vi "Read_BIn.vi"(0 "Refnum in":refnum<k21>, 5 "error in (no error)":errorcluster) -> (14 "Refnum out":refnum<k21>, 15 "Estados":bool[](array[boolean]), 19 "error out":errorcluster)   [LabVIEW 2013]
uses:
  <vilib>/DAQmx/read.llb/DAQmx Read (Digital U32 1Chan 1Samp).vi
  <vilib>/DAQmx/miscellaneous.llb/DAQmx Fill In Error Info.vi
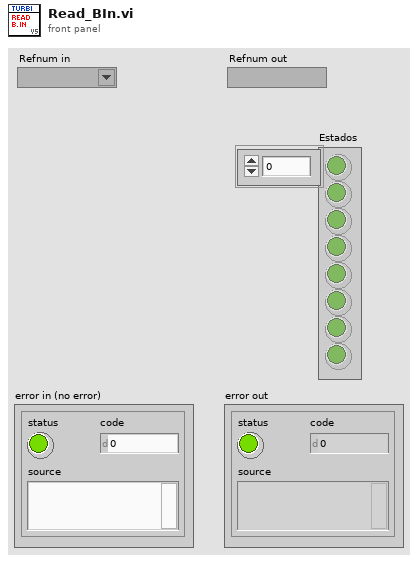
[diagram p1: front panel]
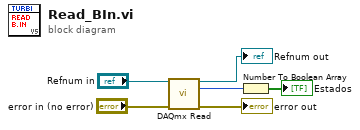
[diagram p0: block diagram]
diagram:
  n1 = call-poly <vilib>:"DAQmx Read.vi"("task/channels in"="Refnum in", "error in"="error in (no error)") -> ("task out"=→"Refnum out":refnum<k21>, "data"=w6:u32, "error out"=→"error out":errorcluster)  [unwired: 11 in]
  n2 = Number To Boolean Array(number=w6) -> (Boolean array=→"Estados":bool[])
